vi "Error站_Leader.vi"(8 "error in":errorcluster) -> (0 "error out":errorcluster)   [LabVIEW 2015]
panel:
  out "ref out":T1
  in  "ref in":T1
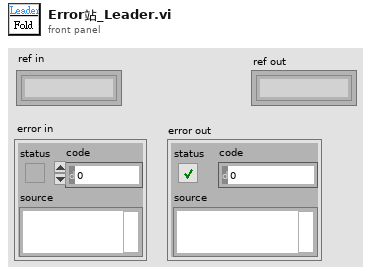
[diagram p1: front panel]
types:
  T1 = typedef "Error站_ref.ctl" = refnum<k1>
  T2 = typedef "Error站_Flag.ctl" = cluster{"0":bool, "1":bool, "2":bool, "3":bool, "4":bool, "5":bool, "6":bool, "7":bool, "8":bool, "9":bool, "10":bool, "11":bool, "12":bool, "13":bool, "14":bool, "15":bool, "16":bool, "17":bool, "18":bool, "19":bool, "20":bool, "21":bool, "22":bool, "23":bool, "24":bool, "25":bool, "26":bool, "27":bool, "28":bool, "29":bool}
  T3 = typedef "Error站_Mode.ctl" = enum8{"Idle", "Run", "Pause", "Err"}
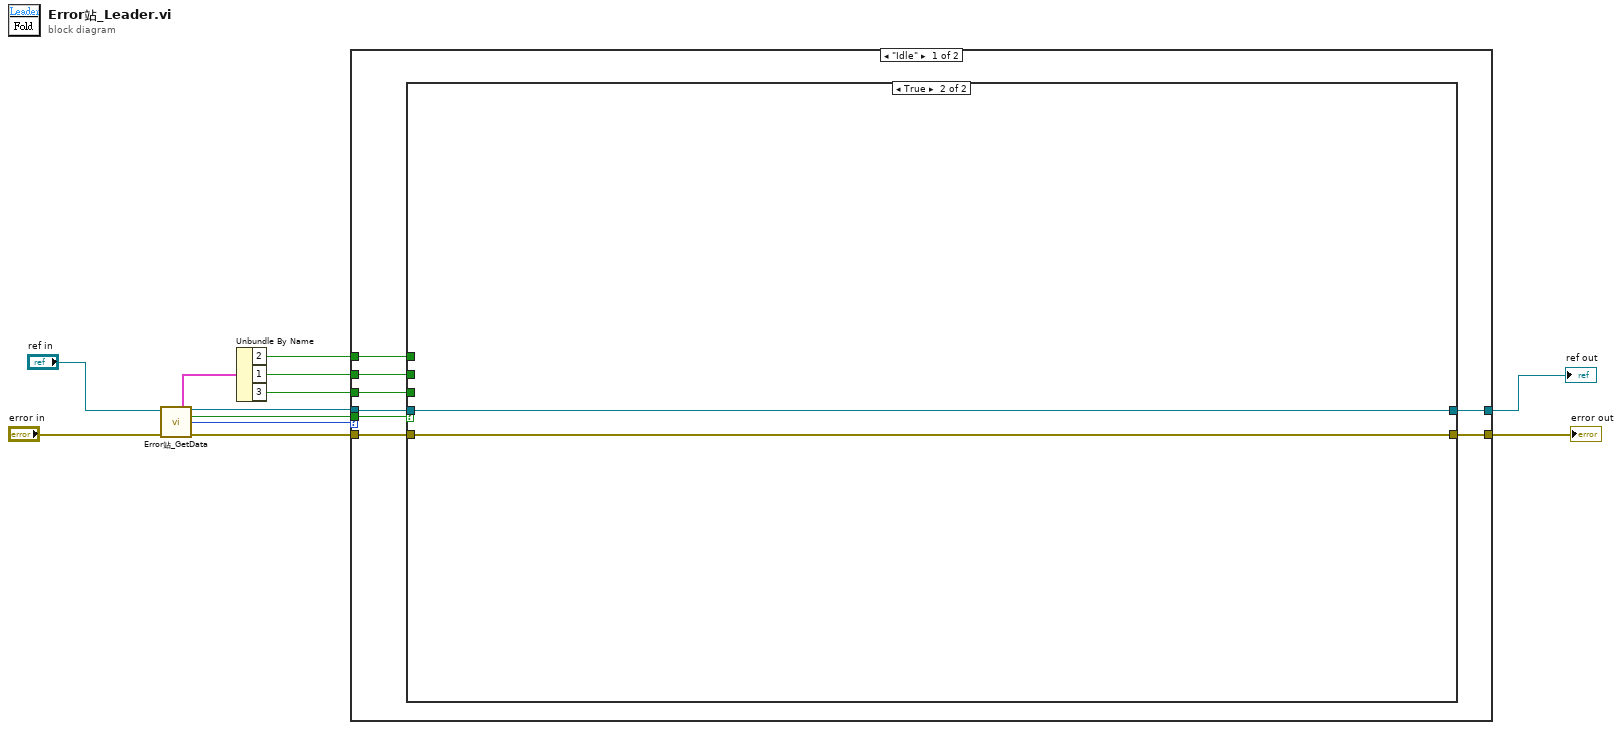
[diagram p0: block diagram]
diagram:
  n1 = call "Error站_GetData.vi"("ref in"="ref in", "error in"="error in") -> ("Flag out"=w11:T2, "ref out"=w9:T1, "Ready"=w6:bool, "Mode"=w10:T3, "error out"=w8:errorcluster)  [unwired: 7 in, 2 out]
  n2 = Unbundle By Name(w11) -> ("2"=w4:bool, "1"=w5:bool, "3"=w1:bool)
  n3 = case shown="\"Idle\"" w10 {
    tunnel: w9 -> [w19 w25]
    tunnel: w8 -> [w17 w26]
    tunnel: [w18 w26] -> w7
    tunnel: [w20 w25] -> w2
    tunnel: w6 -> [w16 _]
    tunnel: w1 -> [w15 _]
    tunnel: w5 -> [w14 _]
    tunnel: w4 -> [w13 _]
    frame "Idle" {
      n4 = case shown="True" w16 {
        tunnel: [w21 w24] -> w20
        tunnel: w19 -> [w21 w24]
        tunnel: [w22 w23] -> w18
        tunnel: w17 -> [w22 w23]
        tunnel: w15 -> [_ _]
        tunnel: w14 -> [_ _]
        tunnel: w13 -> [_ _]
        frame False {
        }
        frame True {
        }
      }
    }
    frame "Run", Default {
    }
  }
  "error out" <- w7
  "ref out" <- w2
